vi "Patrick-multichannel-Sim-Aq.vi"(4 "Cluster":T1={"1/f vs. Uniform "=1.0, "DC Drift Fraction"=0.0, "DC Drift Freq"=0.19999999999999996, "DC Offset"=0.0, "60Hz Amplitude"=0.005, "Gauss/Unif %"=0.5, "Sig Amp"=1.0, "Noise Amp"=0.005} {"Noise Amp" format="%.1p"; "Sig Amp" format="%.2p"; "Gauss/Unif %" min=0.0 max=1.0 step=0.05 format="%.2f"; "60Hz Amplitude" min=0.0 max=10.0 step=0.05 format="%.2p"; "DC Offset" min=-1.0 max=1.0 step=0.01 format="%.2f"; "DC Drift Freq" min=0.0 max=5.0 step=0.05 format="%.2f"; "DC Drift Fraction" format="%.2f"; "1/f vs. Uniform" min=0.0 max=50.0 step=0.5 format="%.1p"}, 5 "Data":waveform(dbl)[][](array[waveform]), 6 "sampling info":cluster{"Fs":dbl, "#s":dbl}={"Fs"=204800.0, "#s"=20480.0}) -> (0 "Data":waveform(dbl)[](array[waveform]))   [LabVIEW 2016, in "LockinDAQ.lvclass"]
uses:
  LockinDAQ.lvclass
  <vilib>/Analysis/2dsp.llb/Real FFT.vi
  <vilib>/Analysis/2dsp.llb/Inverse Real FFT.vi
  <vilib>/Analysis/3filter.llb/Butterworth Filter (DBL).vi
  <vilib>/measure/NI_MABase.lvlib
  <vilib>/Analysis/NI_AALPro.lvlib
  <vilib>/Analysis/NI_AALBase.lvlib
panel:
  out "Waveform Graph":waveform(dbl)[](graph)
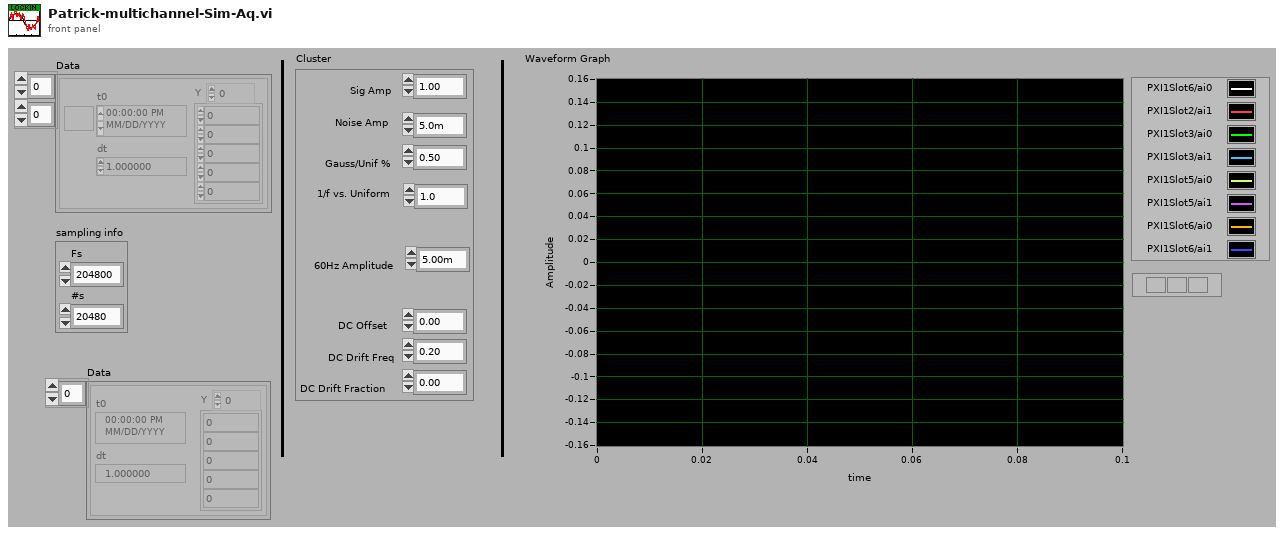
[diagram p1: front panel]
types:
  T1 = cluster{"1/f vs. Uniform ":dbl, "DC Drift Fraction":dbl, "DC Drift Freq":dbl, "DC Offset":dbl, "60Hz Amplitude":dbl, "Gauss/Unif %":dbl, "Sig Amp":dbl, "Noise Amp":dbl}
  T2 = enum32{"Lowpass", "Highpass", "Bandpass", "Bandstop"}
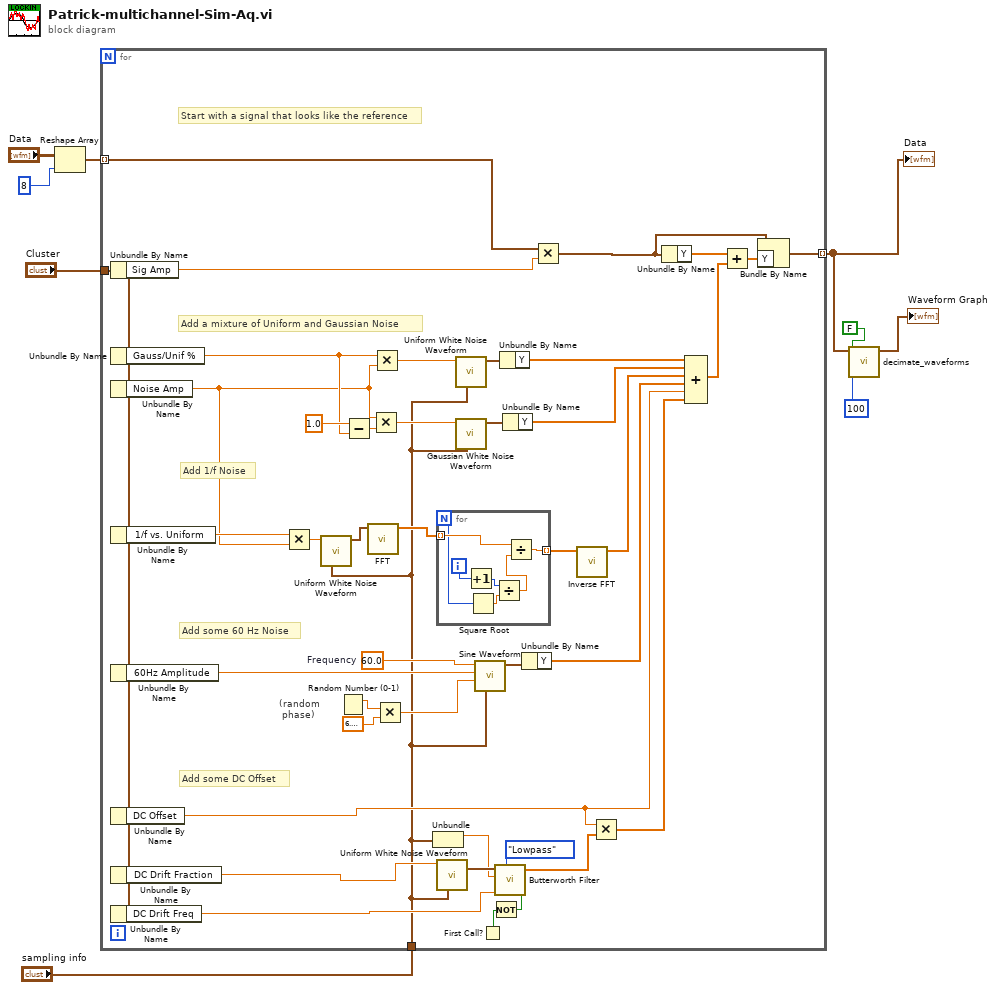
[diagram p0: block diagram]
diagram:
  n1 = Reshape Array("Data", 8 ("dimension size")) -> (w5:waveform(dbl)[])
  n2 = for {
    tunnel: "Cluster" -> [w19]
    tunnel: "sampling info" -> [w16]
    tunnel: w5 -> [w14] mode=indexing
    tunnel: [w10] -> w2 mode=indexing
    w45 = 60.0  # Frequency
    # "Start with a signal that looks like the reference"
    # "Add 1/f Noise"
    # "(random\n phase)"
    # "Add some DC Offset"
    # "Add some 60 Hz Noise"
    # "Add a mixture of Uniform and Gaussian Noise"
    n3 = Unbundle By Name(w19) -> ("Sig Amp"=w15:dbl)
    n4 = Unbundle By Name(w19) -> ("Gauss/Unif %"=w24:dbl)
    n5 = Unbundle By Name(w19) -> ("Noise Amp"=w22:dbl)
    n6 = Unbundle By Name(w19) -> ("1/f vs. Uniform"=w23:dbl)
    n7 = Unbundle By Name(w19) -> ("60Hz Amplitude"=w21:dbl)
    n8 = Unbundle By Name(w19) -> ("DC Offset"=w20:dbl)
    n9 = Unbundle By Name(w19) -> ("DC Drift Fraction"=w17:dbl)
    n10 = Unbundle By Name(w19) -> ("DC Drift Freq"=w18:dbl)
    n11 = Multiply(x=w23, y=w22) -> (x*y=w32:dbl)
    n12 = call <vilib>:"Uniform White Noise Waveform.vi"("sampling info"=w16, "amplitude"=w32) -> ("signal out"=w31:waveform(dbl))  [unwired: 8 in, 1 out]
    n13 = Random Number (0-1)() -> (number: 0 to 1=w43:dbl)
    n14 = Subtract(x=1.0, y=w24) -> (x-y=w47:dbl)
    n15 = call-poly <vilib>:"FFT.vi"("X"=w31) -> ("FFT {X}"=w34:cdb[])  [unwired: 9 in, 1 out]
    n16 = Multiply(x=w22, y=w47) -> (x*y=w49:dbl)
    n17 = Multiply(x=w24, y=w22) -> (x*y=w48:dbl)
    n18 = Multiply(x=w43, y=6.283185307179586) -> (x*y=w42:dbl)
    n19 = Unbundle(w16) -> ("Fs"=w39:dbl)  [unwired: 1 out]
    n20 = for {
      N -> [w55]
      tunnel: [w58] -> w33 mode=indexing
      tunnel: w34 -> [w57] mode=indexing
      i -> [w56]
      n21 = Increment(x=w56) -> (x+1=w53:i32)
      n22 = Square Root(x=w55) -> (sqrt(x)=w54:dbl)
      n23 = Divide(x=w53, y=w54) -> (x/y=w52:dbl)
      n24 = Divide(x=w57, y=w52) -> (x/y=w58:cdb)
    }
    n25 = call <vilib>:"Uniform White Noise Waveform.vi"("sampling info"=w16, "amplitude"=w17) -> ("signal out"=w40:waveform(dbl))  [unwired: 8 in, 1 out]
    n26 = call <vilib>:"Uniform White Noise Waveform.vi"("sampling info"=w16, "amplitude"=w48) -> ("signal out"=w50:waveform(dbl))  [unwired: 8 in, 1 out]
    n27 = call <vilib>:"Gaussian White Noise Waveform.vi"("sampling info"=w16, "standard deviation"=w49) -> ("signal out"=w51:waveform(dbl))  [unwired: 8 in, 1 out]
    n28 = call <vilib>:"Sine Waveform.vi"("sampling info"=w16, "phase"=w42, "amplitude"=w21, "frequency"=w45) -> ("signal out"=w41:waveform(dbl))  [unwired: 6 in, 1 out]
    n29 = First Call?() -> (First Call?: T/F=w25:bool)
    n30 = Not(x=w25) -> (.not. x?=w37:bool)
    n31 = call-poly <vilib>:"Butterworth Filter.vi"("init/cont (init:F)"=w37, "filter type"=T2."Lowpass", "low cutoff freq: fl"=w18, "sampling freq: fs"=w39, "X"=w40) -> ("Filtered X"=w36:dbl[])  [unwired: 3 in, 1 out]
    n32 = Unbundle By Name(w50) -> ("Y"=w35:dbl[])
    n33 = Unbundle By Name(w51) -> ("Y"=w26:dbl[])
    n34 = Unbundle By Name(w41) -> ("Y"=w30:dbl[])
    n35 = Multiply(x=w14, y=w15) -> (x*y=w11:waveform(dbl))
    n36 = call-poly <vilib>:"Inverse FFT.vi"("FFT {X}"=w33) -> ("X"=w29:dbl[])  [unwired: 9 in, 1 out]
    n37 = Multiply(x=w20, y=w36) -> (x*y=w28:dbl[])
    n38 = Unbundle By Name(w11) -> ("Y"=w13:dbl[])
    n39 = Compound Arithmetic op=ADD(w35, w26, w29, w30, w20, w28) -> (w27:dbl[])
    n40 = Add(x=w13, y=w27) -> (x+y=w12:dbl[])
    n41 = Bundle By Name(cluster=w11, "Y"=w12) -> (w10:waveform(dbl))
  }
  "Data" <- w2
  n42 = call "decimate_waveforms.vi"("Input Signal"=w2, "averaging"=FALSE, "decimating factor"=100) -> ("Decimated Waveforms"=→"Waveform Graph":waveform(dbl)[])  [unwired: 6 in, 1 out]
